vi "Convert to meters.vi"(1 "Lithography Data In":T1(array[cluster])) -> (0 "Lithography Data Out":T1(array[cluster]))   [LabVIEW 2016]
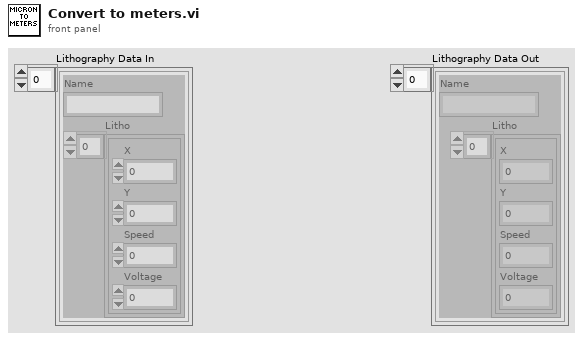
[diagram p1: front panel]
types:
  T1 = cluster{"Name":string, "Litho":cluster{"X":dbl, "Y":dbl, "Speed":dbl, "Voltage":dbl}[]}[]
  T2 = cluster{"X":dbl, "Y":dbl, "Speed":dbl, "Voltage":dbl}[]
  T3 = cluster{"X":dbl, "Y":dbl, "Speed":dbl, "Voltage":dbl}
  T4 = cluster{"Name":string, "Litho":cluster{"X":dbl, "Y":dbl, "Speed":dbl, "Voltage":dbl}[]}
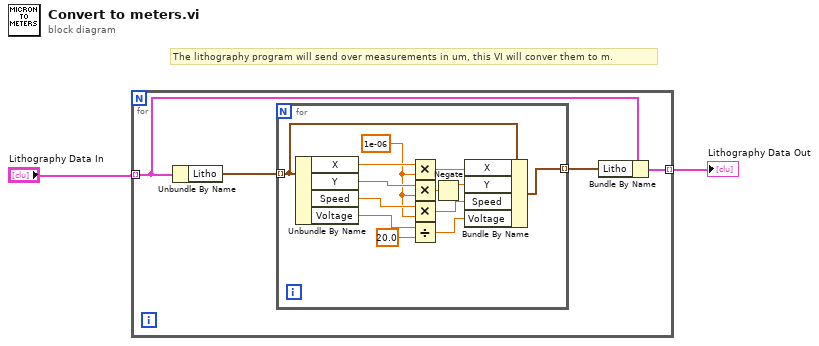
[diagram p0: block diagram]
diagram:
  # "The lithography program will send over measurements in um, this VI will conver them to m."
  n1 = for {
    tunnel: "Lithography Data In" -> [w5] mode=indexing
    tunnel: [w4] -> w2 mode=indexing
    n2 = Unbundle By Name(w5) -> ("Litho"=w6:T2)
    n3 = for {
      tunnel: w6 -> [w15] mode=indexing
      tunnel: [w14] -> w3 mode=indexing
      w16 = 1e-06 ("y")
      n4 = Unbundle By Name(w15) -> ("X"=w19:dbl, "Y"=w17:dbl, "Speed"=w18:dbl, "Voltage"=w9:dbl)
      n5 = Multiply(x=w19, y=w16) -> (x*y=w13:dbl)
      n6 = Multiply(x=w17, y=w16) -> (x*y=w12:dbl)
      n7 = Multiply(x=w18, y=w16) -> (x*y=w11:dbl)
      n8 = Divide(x=w9, y=20.0) -> (x/y=w7:dbl)
      n9 = Negate(x=w12) -> (-x=w10:dbl)
      n10 = Bundle By Name(cluster=w15, "X"=w13, "Y"=w10, "Speed"=w11, "Voltage"=w7) -> (w14:T3)
    }
    n11 = Bundle By Name(cluster=w5, "Litho"=w3) -> (w4:T4)
  }
  "Lithography Data Out" <- w2
